vi "Get Array of Pos frontend.vi"(8 "error in (no error)":errorcluster, 11 "Motions in":refnum<class "Motions.lvclass">) -> (0 "error out":errorcluster, 2 "Array of pos frontend":dbl[](array[numeric]), 3 "Motions out":refnum<class "Motions.lvclass">)   [LabVIEW 2016, in "Hardware.lvlib" / "Motions.lvlib" / "Motions.lvclass"]
uses:
  <userlib>/Common Components/Hardware/Abstract System/Motions/Motions/Motions.lvclass
  <userlib>/Common Components/Hardware/Abstract System/Motions/Motions/Motions.lvclass/Motions.ctl
  <userlib>/Common Components/Hardware/Motor/Motor/Motor.lvclass
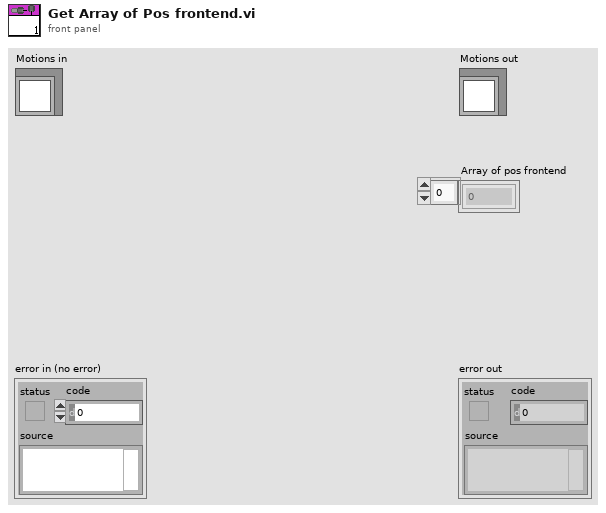
[diagram p1: front panel]
types:
  T1 = cluster{"Connected":bool, "Enabled":bool, "Moving Status":bool, "Soft Moving Status":bool, "Current Pos":dbl, "Target Pos":dbl, "Moving Dir (-1, 0, 1)":i32, "Error Status":bool, "Hard Limit+":bool, "Hard Limit-":bool, "Soft Limit+":bool, "Soft Limit-":bool}[]
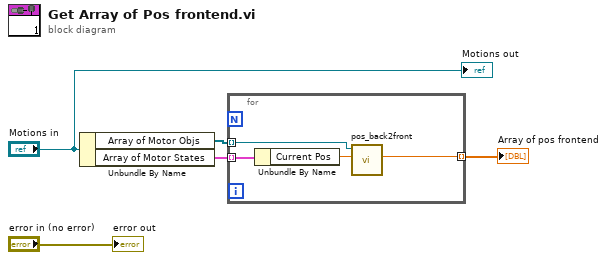
[diagram p0: block diagram]
diagram:
  n1 = Unbundle By Name("Motions in") -> ("Array of Motor Objs"=w3:refnum<class "Motor.lvclass">[], "Array of Motor States"=w2:T1)
  n2 = for {
    tunnel: w3 -> [w8] mode=indexing
    tunnel: w2 -> [w9] mode=indexing
    tunnel: [w6] -> w1 mode=indexing
    n3 = Unbundle By Name(w9) -> ("Current Pos"=w7:dbl)
    n4 = call <userlib>:"pos_back2front.vi"("pos backend"=w7, "Motor in"=w8) -> ("pos frontend"=w6:dbl)  [unwired: 7 in, 2 out]
  }
  "Array of pos frontend" <- w1
  "error out" <- "error in (no error)"
  "Motions out" <- "Motions in"
